vi "TestObservePath_ValueCFolderFileDotExt.vi"(8 "error in (no error)":errorcluster, 11 "TestCase in":refnum<class "TestObservableData.lvclass">) -> (0 "error out":errorcluster, 3 "TestCase out":refnum<class "TestObservableData.lvclass">)   [LabVIEW 2015, in "TestObservableData.lvclass"]
uses:
  TestObservableData.lvclass
  TestObservableData.lvclass/TestObservableData.ctl
  Framework/SubscriptionPolicy/BasicSubscription/BasicSubscription.lvclass/BasicSubscription.ctl
  Framework/IMediator/SubscriptionRequest/SubscriptionRequest.lvclass/SubscriptionRequest.ctl
  Framework/IMediator/IMediator Messages/Subscribe Msg/Subscribe Msg.lvclass/Subscribe Msg.ctl
  <vilib>/ActorFramework/Message Enqueuer/Message Enqueuer.lvclass/Message Enqueuer.ctl
  <vilib>/ActorFramework/Message Enqueuer/Enqueue.vi
  <vilib>/ActorFramework/Message Priority Queue/Priority Enqueue.vi
  Framework/SubscriptionPolicy/BasicSubscription/BasicSubscription.lvclass
  Framework/IMediator/SubscriptionRequest/SubscriptionRequest.lvclass
  Framework/IMediator/IMediator Messages/Subscribe Msg/Subscribe Msg.lvclass
  Framework/IMediator/ISubscriptionPolicy/ISubscriptionPolicy.lvclass
  Framework/Transport/TerminalBinding/TerminalBinding.lvclass
panel:
  out "ControlTerminal":path
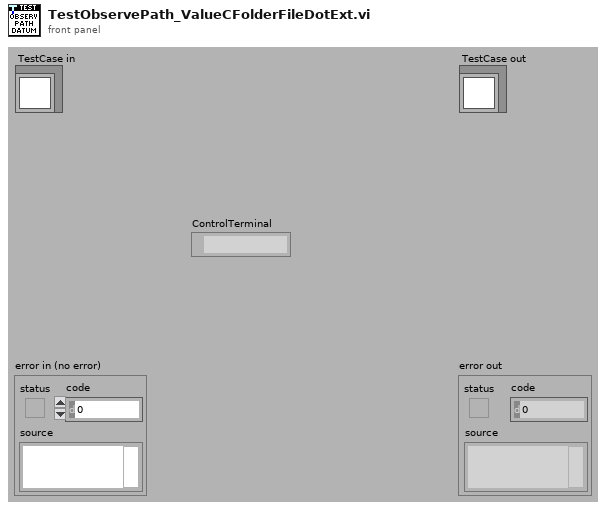
[diagram p1: front panel]
types:
  T1 = typedef "IMediator.lvlib/ISubscriptionPolicy.lvclass/ISubscriptionPolicy Reference.ctl" = refnum<data-value>
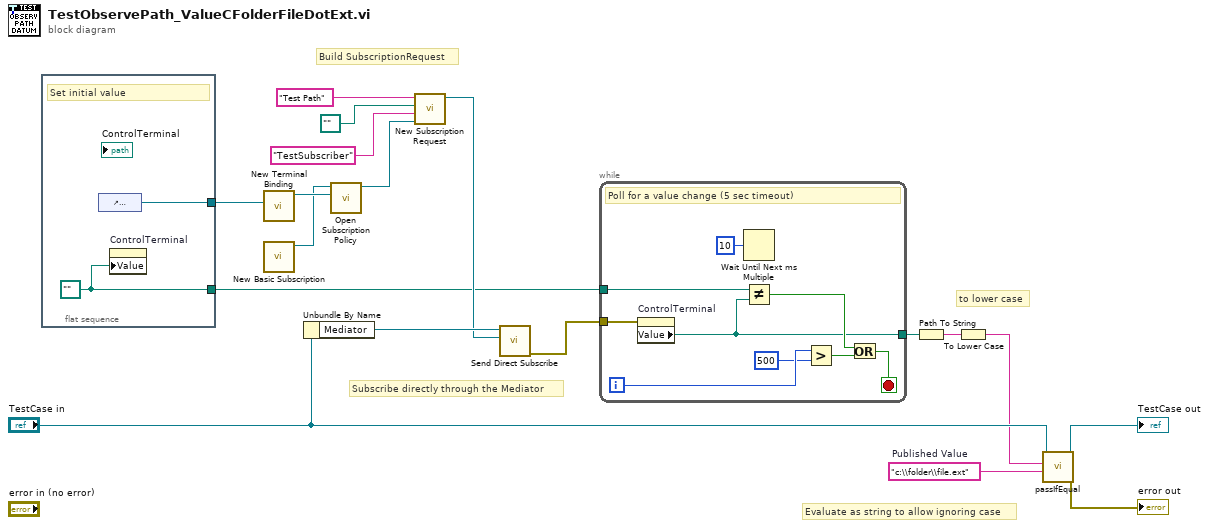
[diagram p0: block diagram]
diagram:
  w4 = "c:\\folder\\file.ext"  # Published Value
  # "to lower case"
  # "Evaluate as string to allow ignoring case"
  # "Build SubscriptionRequest"
  # "Subscribe directly through the Mediator"
  n1 = flat-sequence {
    tunnel: [w20] -> w8
    tunnel: [w19] -> w6
    frame #0 {
      w19 = path "" ("ControlTerminal")
      # "Set initial value"
      n2 = control-ref of="ControlTerminal"() -> (w20:refnum<vi>)
      n3 = property on="ControlTerminal" class="Path"("Value"=w19) -> ()  [unwired: 2 in, 2 out]
    }
  }
  n4 = call "New Terminal Binding.vi"("Ctl Refnum"=w8) -> ("TerminalBinding"=w9:refnum<class "TerminalBinding.lvclass">)  [unwired: 9 in, 1 out]
  n5 = call "New Basic Subscription.vi"() -> ("BasicSubscription Out"=w1:refnum<class "BasicSubscription.lvclass">)  [unwired: 11 in]
  n6 = Unbundle By Name("TestCase in") -> ("Mediator"=w15:refnum<class "Message Enqueuer.lvclass">)
  n7 = call "Open Subscription Policy.vi"("Transport"=w9, "SubscriptionPolicy"=w1) -> ("Subscription Policy"=w10:T1)  [unwired: 8 in, 1 out]
  n8 = call "New Subscription Request.vi"("Subscription Policy"=w10, "Subscriber ID"="TestSubscriber" ("Unique Subscriber ID"), "Type"=path "", "Datum Name"="Test Path" ("Topic Name")) -> ("SubscriptionRequest"=w14:refnum<class "SubscriptionRequest.lvclass">)  [unwired: 7 in]
  n9 = call "Send Direct Subscribe.vi"("Subscription Request"=w14, "Message Enqueuer"=w15) -> ("error out"=w7:errorcluster)  [unwired: 8 in, 1 out]
  n10 = while {
    tunnel: w7 -> [w29]
    tunnel: w6 -> [w28]
    tunnel: [w21] -> w5
    i -> [w24]
    stop <- w22 stop-if-true
    # "Poll for a value change (5 sec timeout)"
    n11 = property on="ControlTerminal" class="Path"(error in=w29) -> ("Value"=w21:path)  [unwired: 1 in, 2 out]
    n12 = Wait Until Next ms Multiple(millisecond multiple=u32 10 ("milliseconds to wait")) -> ()  [unwired: 1 out]
    n13 = Not Equal?(x=w28, y=w21) -> (x != y?=w27:bool)
    n14 = Greater?(x=w24, y=500) -> (0:w25:bool)
    n15 = Or(x=w27, y=w25) -> (x .or. y?=w22:bool)
  }
  n16 = Path To String(path=w5) -> (string=w3:string)
  n17 = To Lower Case(string=w3) -> (all lower case string=w2:string)
  n18 = call-dynamic "passIfEqual.vi"("y"=w4, "x"=w2, "TestCase in"="TestCase in") -> ("error out"=→"error out":errorcluster, "TestCase out"=→"TestCase out":refnum<class "TestObservableData.lvclass">)  [unwired: 7 in]
